vi "Read Screen Tap.vi"   [LabVIEW 2011, in "LMH-Leap.lvlib"]
doc: "Read all data from screen tap gestures. Use the polymorphic instance to select bewteen on and N screen tap gestures."
uses:
  LMH-Leap.lvlib
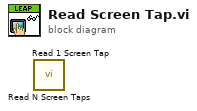
[diagram p0: block diagram]
diagram:
  n1 = call "Read N Screen Taps.vi"() -> ()  [unwired: 8 in, 4 out]
  n2 = call "Read 1 Screen Tap.vi"() -> ()  [unwired: 8 in, 4 out]
